vi "Crossover Frame.vi"(8 "error in (no error)":errorcluster, 10 "OSSP_Problem In":refnum<class "OSSP_Problem.lvclass">, 11 "GA in":refnum<class "GA.lvclass">) -> (0 "error out":errorcluster, 2 "OSSP_Problem Out":refnum<class "OSSP_Problem.lvclass">, 3 "GA out":refnum<class "GA.lvclass">)   [LabVIEW 2013, in "GA.lvclass"]
uses:
  GA.lvclass
  OSSP_Problem.lvclass
  GA.lvclass/GA.ctl
  OSSP_Problem.lvclass/OSSP_Problem.ctl
  Controls/MPOX1 Operation Selection Rule.ctl
  Controls/MPOX2 Operation Selection Rule.ctl
  Find Elements not On Other Child.vi
  GA/SubVIS/Remove Duplicates In Array.vi
  GA/SubVIS/OX Crossover Template.vi
  LOX Crossover Template.vi
  Scheduler_Class/Schedule To Operations on Machines.vi
  OSSP_Problem_Class/Getters/Read Processing Times.vi
  Calculate Job and Machine Orders.vi
  Getters/Read Scheduler.vi
  Getters/Read Objective .vi
  MOPX1 Engine.vi
  Scheduler_Class/NonDelay Scheduler/Non Delay Scheduler Engine.vi
  Scheduler_Class/Giffler Thompson Active Schedule Engine.vi
  Scheduler_Class/MyFIFOScheduler.vi
  Scheduler_Class/Job Completion Times.vi
  Scheduler_Class/Prins FIFO Scheduler Methods and Controls/Prins FIFO Scheduler.vi
  Scheduler_Class/Prins FIFO Scheduler Methods and Controls/Methods/Calculate Final Completion Times of Jobs.vi
  OSSP_Problem_Class/Getters/Read Due Dates.vi
  MOPX2 Engine.vi
  Scheduler_Class/Operation to Machine Job Tuple.vi
  Scheduler_Class/Check Other Machines for Schedule Time.vi
  Scheduler_Class/Schedule Job.vi
  Scheduler_Class/Find Gaps on Particular Machine.vi
  Scheduler_Class/Increment Number of Jobs on Machine.vi
  Scheduler_Class/Find Job On Other Machines.vi
  Scheduler_Class/Prins FIFO Scheduler Methods and Controls/Methods/UpdateMachineGaps.vi
  Scheduler_Class/Prins FIFO Scheduler Methods and Controls/Methods/UpdateJobGaps.vi
  Scheduler_Class/Prins FIFO Scheduler Methods and Controls/Methods/Find Intersecting Gaps.vi
  Scheduler_Class/GT Algorithm Find M_ok and J_ok.vi
  Scheduler_Class/Prins FIFO Scheduler Methods and Controls/Methods/Transform to Plain Job and Machine Gaps Array.vi
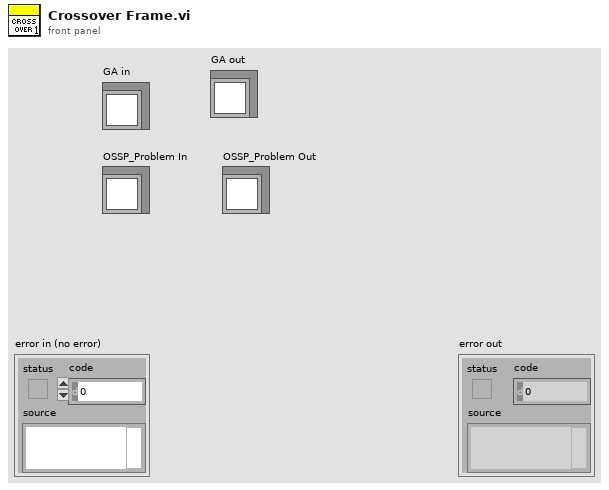
[diagram p1: front panel]
types:
  T1 = typedef "GA.lvclass/MPOX1 Operation Selection Rule.ctl" = enum16{"Min Lateness Job", "Random Job"}
  T2 = typedef "GA.lvclass/MPOX2 Operation Selection Rule.ctl" = enum16{"First Operation of All Jobs", "Random"}
  T3 = typedef "Solution_GA.ctl" = cluster{"Schedule":u16[], "Fitness":u16, "Fitness Valid?":bool}
  T4 = typedef "GA.lvclass/Crossover Type.ctl" = enum16{"One Point Cx", "Two Point Cx", "Ordered Cx (OX)", "Linear Order Cx (LOX)", "PMX", "Uniform PMX", "Cycle Cx", "Specialized Cx", "JO4M Cx", "MPOX1", "MPOX1 Random", "MPOX2", "MPOX2 Random", "SXX"}
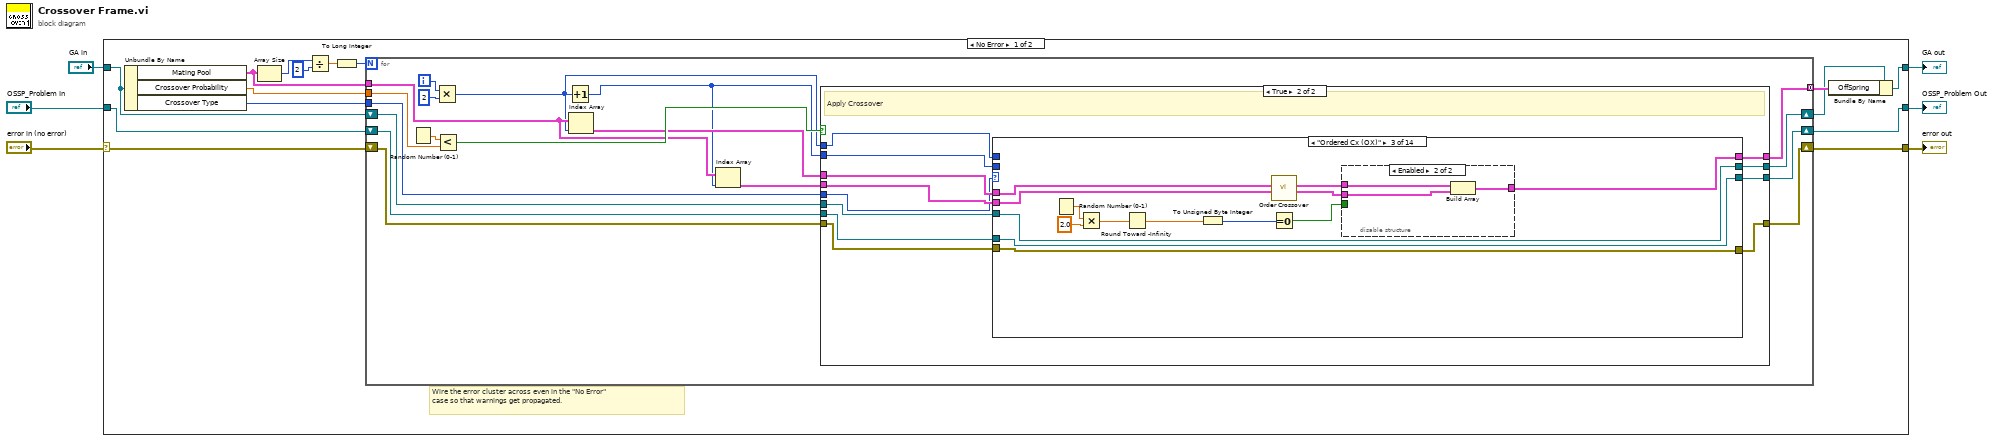
[diagram p0: block diagram]
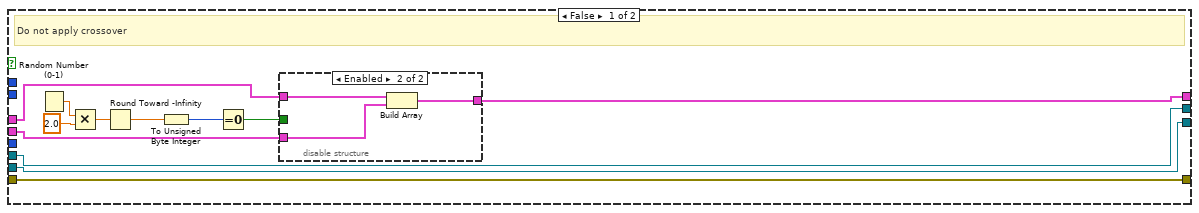
[diagram p2: hidden frame]
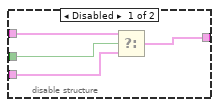
[diagram p3: hidden frame]
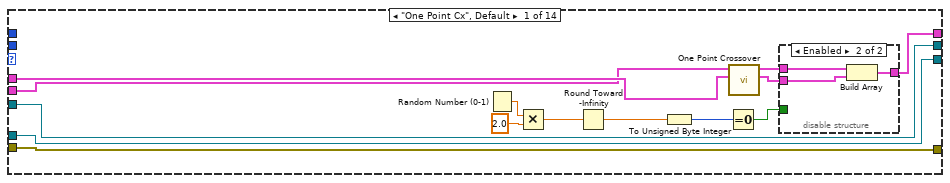
[diagram p4: hidden frame]
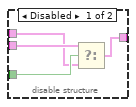
[diagram p5: hidden frame]
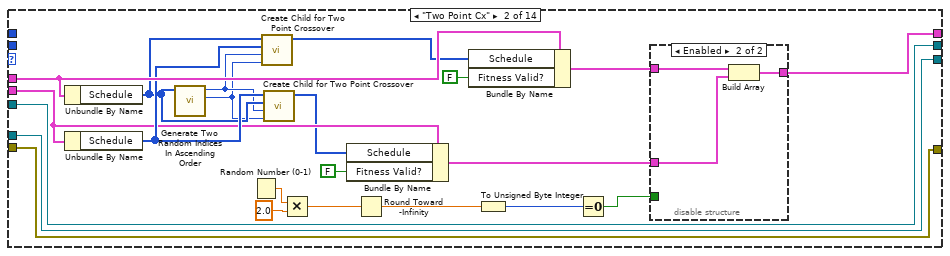
[diagram p6: hidden frame]
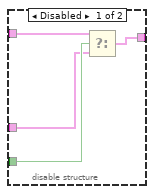
[diagram p7: hidden frame]
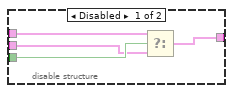
[diagram p8: hidden frame]
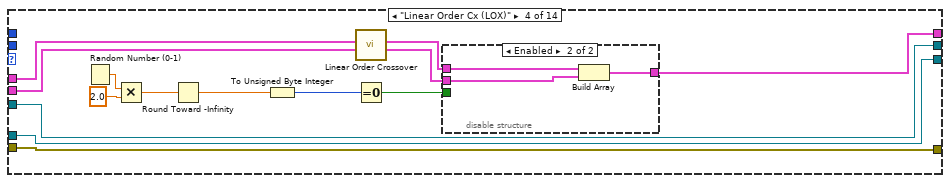
[diagram p9: hidden frame]
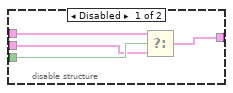
[diagram p10: hidden frame]
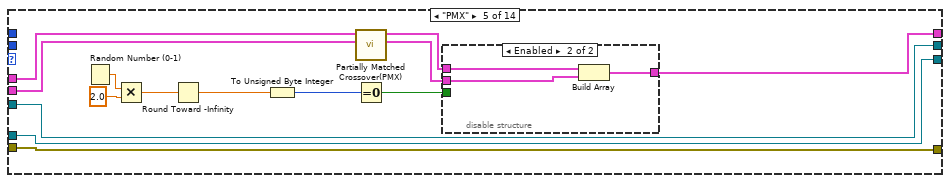
[diagram p11: hidden frame]
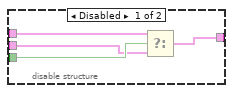
[diagram p12: hidden frame]
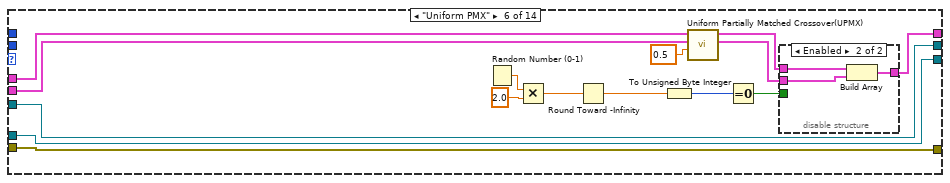
[diagram p13: hidden frame]
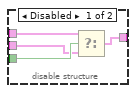
[diagram p14: hidden frame]
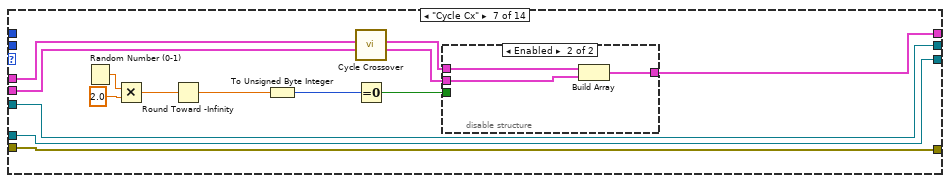
[diagram p15: hidden frame]
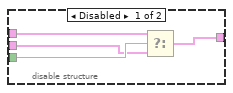
[diagram p16: hidden frame]
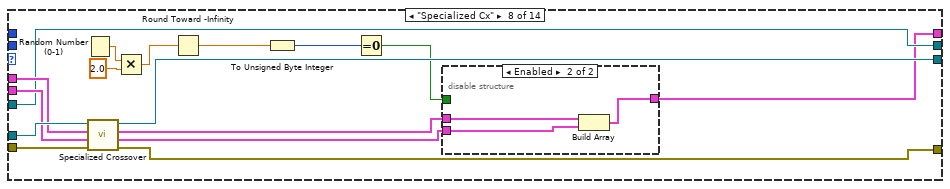
[diagram p17: hidden frame]
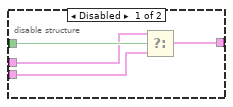
[diagram p18: hidden frame]
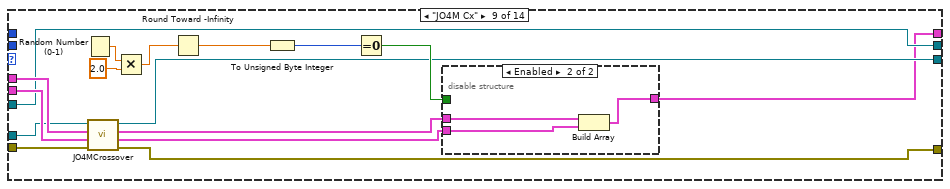
[diagram p19: hidden frame]
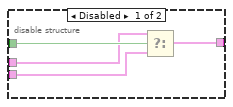
[diagram p20: hidden frame]
diagram:
  n1 = case shown="No Error" "error in (no error)" {
    selector: "error in (no error)" -> [w15 w410]
    tunnel: [w14 w410] -> w5
    tunnel: [w19 w409] -> w3
    tunnel: "GA in" -> [w8 w409]
    tunnel: "OSSP_Problem In" -> [w17 w408]
    tunnel: [w16 w408] -> w1
    frame No Error {
      # "Wire the error cluster across even in the \"No Error\"\ncase so that warnings get propagated."
      n2 = Unbundle By Name(w8) -> ("Mating Pool"=w21:T3[], "Crossover Probability"=w20:dbl, "Crossover Type"=w18:T4)
      n3 = Array Size(array=w21) -> (size(s)=w13:i32)
      n4 = Divide(x=w13, y=2) -> (x/y=w9:dbl)
      n5 = To Long Integer(number=w9) -> (32bit integer=w12:i32)
      n6 = for {
        N: w12 -> [_]
        tunnel: w20 -> [w37]
        tunnel: w18 -> [w30]
        shift-right: [w29] -> w16
        shift-left: w17 -> [w28]
        shift-right: [w26] -> w14
        shift-left: w15 -> [w27]
        tunnel: w21 -> [w33]
        tunnel: [w24] -> w11 mode=concatenating
        shift-right: [w22] -> w7
        shift-left: w8 -> [w23]
        i -> [w39]
        n7 = Random Number (0-1)() -> (number: 0 to 1=w38:dbl)
        n8 = Multiply(x=w39, y=2) -> (x*y=w32:i32)
        n9 = Less?(x=w38, y=w37) -> (x < y?=w36:bool)
        n10 = Increment(x=w32) -> (x+1=w31:i32)
        n11 = Index Array(array=w33, index=w32) -> (element=w35:T3)
        n12 = Index Array(array=w33, index=w31) -> (element=w34:T3)
        n13 = case shown="True" w36 {
          tunnel: w35 -> [w43 w68]
          tunnel: w34 -> [w42 w67]
          tunnel: w32 -> [_ w70]
          tunnel: w31 -> [_ w69]
          tunnel: w30 -> [_ w66]
          tunnel: w28 -> [w51 w65]
          tunnel: [w51 w64] -> w29
          tunnel: w27 -> [w50 w63]
          tunnel: [w50 w62] -> w26
          tunnel: [w40 w61] -> w24
          tunnel: w23 -> [w41 w60]
          tunnel: [w41 w59] -> w22
          frame False {
            # "Do not apply crossover"
            n14 = Random Number (0-1)() -> (number: 0 to 1=w49:dbl)
            n15 = Multiply(x=w49, y=2.0) -> (x*y=w47:dbl)
            n16 = Round Toward -Infinity(1:w47) -> (0:w46:dbl)
            n17 = To Unsigned Byte Integer(number=w46) -> (unsigned 8bit integer=w45:u8)
            n18 = Equal To 0?(x=w45) -> (x = 0?=w44:bool)
            n19 = disable-structure shown="Enabled" {
              disable-tunnel: w44 -> [w55 _]
              disable-tunnel: w43 -> [w54 w58]
              disable-tunnel: w42 -> [w53 w57]
              disable-tunnel: [w52 w56] -> w40
              frame Disabled {
                n20 = Select(t=w54, s=w55, f=w53) -> (s? t:f=w52:T3)
              }
              frame Enabled {
                n21 = Build Array(w58, w57) -> (w56:T3[])
              }
            }
          }
          frame True {
            # "Apply Crossover"
            n22 = case shown="\"Ordered Cx (OX)\"" w66 {
              tunnel: w70 -> [_ _ _ _ _ _ _ _ _ _ _ _ _ _]
              tunnel: w69 -> [_ _ _ _ _ _ _ _ _ _ _ _ _ _]
              tunnel: w68 -> [w84 w111 w132 w153 w173 w194 w217 w237 w259 w289 w316 w344 w370 w400]
              tunnel: w67 -> [w83 w104 w131 w152 w172 w193 w216 w238 w258 w288 w315 w343 w369 w399]
              tunnel: w65 -> [w82 w113 w133 w154 w176 w198 w219 w242 w257 w285 w312 w333 w359 w383]
              tunnel: [w82 w113 w133 w154 w176 w198 w219 w241 w254 w284 w311 w330 w356 w382] -> w64
              tunnel: w63 -> [w81 w112 w134 w155 w175 w197 w218 w240 w256 w292 w319 w345 w371 w386]
              tunnel: [w81 w112 w134 w155 w175 w197 w218 w239 w255 w283 w310 w341 w367 w385] -> w62
              tunnel: [w71 w92 w121 w142 w163 w184 w206 w227 w250 w273 w300 w327 w353 w379] -> w61
              tunnel: w60 -> [w72 w93 w122 w143 w174 w196 w207 w228 w251 w291 w318 w334 w360 w391]
              tunnel: [w72 w93 w122 w143 w174 w196 w207 w228 w251 w290 w317 w334 w360 w391] -> w59
              frame "One Point Cx", Default {
                n23 = Random Number (0-1)() -> (number: 0 to 1=w80:dbl)
                n24 = Multiply(x=w80, y=2.0) -> (x*y=w78:dbl)
                n25 = Round Toward -Infinity(1:w78) -> (0:w77:dbl)
                n26 = To Unsigned Byte Integer(number=w77) -> (unsigned 8bit integer=w76:u8)
                n27 = Equal To 0?(x=w76) -> (x = 0?=w75:bool)
                n28 = call "One Point Crossover.vi"("Parent 1 in"=w84, "Parent 2 in"=w83) -> ("Child 1 out"=w74:T3, "Child 2 Out"=w73:T3)  [unwired: 8 in]
                n29 = disable-structure shown="Enabled" {
                  disable-tunnel: w75 -> [w88 _]
                  disable-tunnel: w74 -> [w87 w89]
                  disable-tunnel: w73 -> [w86 w91]
                  disable-tunnel: [w85 w90] -> w71
                  frame Disabled {
                    n30 = Select(t=w87, s=w88, f=w86) -> (s? t:f=w85:T3)
                  }
                  frame Enabled {
                    n31 = Build Array(w91, w89) -> (w90:T3[])
                  }
                }
              }
              frame "Two Point Cx" {
                n32 = Unbundle By Name(w111) -> ("Schedule"=w107:u16[])
                n33 = Unbundle By Name(w104) -> ("Schedule"=w108:u16[])
                n34 = call "Generate Two Random Indices In Ascending Order.vi"("Schedule"=w107) -> ("Index 2"=w105:i32, "Index 1"=w106:i32)  [unwired: 9 in]
                n35 = Random Number (0-1)() -> (number: 0 to 1=w101:dbl)
                n36 = call "Create Child for Two Point Crossover.vi"("Cut Point Index 2"=w105, "Cut Point Index 1"=w106, "SCH 2"=w108, "SCH 1"=w107) -> ("Child Out"=w110:u16[])  [unwired: 7 in]
                n37 = call "Create Child for Two Point Crossover.vi"("Cut Point Index 2"=w105, "Cut Point Index 1"=w106, "SCH 2"=w107, "SCH 1"=w108) -> ("Child Out"=w103:u16[])  [unwired: 7 in]
                n38 = Multiply(x=w101, y=2.0) -> (x*y=w99:dbl)
                n39 = Bundle By Name(cluster=w104, "Schedule"=w103, "Fitness Valid?"=FALSE) -> (w94:T3)
                n40 = Round Toward -Infinity(1:w99) -> (0:w98:dbl)
                n41 = Bundle By Name(cluster=w111, "Schedule"=w110, "Fitness Valid?"=FALSE) -> (w95:T3)
                n42 = To Unsigned Byte Integer(number=w98) -> (unsigned 8bit integer=w97:u8)
                n43 = Equal To 0?(x=w97) -> (x = 0?=w96:bool)
                n44 = disable-structure shown="Enabled" {
                  disable-tunnel: w96 -> [w117 _]
                  disable-tunnel: w95 -> [w116 w120]
                  disable-tunnel: w94 -> [w115 w119]
                  disable-tunnel: [w114 w118] -> w92
                  frame Disabled {
                    n45 = Select(t=w116, s=w117, f=w115) -> (s? t:f=w114:T3)
                  }
                  frame Enabled {
                    n46 = Build Array(w120, w119) -> (w118:T3[])
                  }
                }
              }
              frame "Ordered Cx (OX)" {
                n47 = Random Number (0-1)() -> (number: 0 to 1=w130:dbl)
                n48 = Multiply(x=w130, y=2.0) -> (x*y=w128:dbl)
                n49 = Round Toward -Infinity(1:w128) -> (0:w127:dbl)
                n50 = To Unsigned Byte Integer(number=w127) -> (unsigned 8bit integer=w126:u8)
                n51 = call "Order Crossover.vi"("Parent 2"=w131, "Parent 1"=w132) -> ("Child 2"=w123:T3, "Child 1"=w124:T3)  [unwired: 8 in]
                n52 = Equal To 0?(x=w126) -> (x = 0?=w125:bool)
                n53 = disable-structure shown="Enabled" {
                  disable-tunnel: w125 -> [w138 _]
                  disable-tunnel: w124 -> [w137 w141]
                  disable-tunnel: w123 -> [w136 w140]
                  disable-tunnel: [w135 w139] -> w121
                  frame Disabled {
                    n54 = Select(t=w137, s=w138, f=w136) -> (s? t:f=w135:T3)
                  }
                  frame Enabled {
                    n55 = Build Array(w141, w140) -> (w139:T3[])
                  }
                }
              }
              frame "Linear Order Cx (LOX)" {
                n56 = Random Number (0-1)() -> (number: 0 to 1=w151:dbl)
                n57 = Multiply(x=w151, y=2.0) -> (x*y=w149:dbl)
                n58 = Round Toward -Infinity(1:w149) -> (0:w148:dbl)
                n59 = To Unsigned Byte Integer(number=w148) -> (unsigned 8bit integer=w147:u8)
                n60 = call "Linear Order Crossover.vi"("Parent 2"=w152, "Parent 1"=w153) -> ("Child 2"=w144:T3, "Child 1"=w145:T3)  [unwired: 8 in]
                n61 = Equal To 0?(x=w147) -> (x = 0?=w146:bool)
                n62 = disable-structure shown="Enabled" {
                  disable-tunnel: w146 -> [w159 _]
                  disable-tunnel: w145 -> [w158 w162]
                  disable-tunnel: w144 -> [w157 w161]
                  disable-tunnel: [w156 w160] -> w142
                  frame Disabled {
                    n63 = Select(t=w158, s=w159, f=w157) -> (s? t:f=w156:T3)
                  }
                  frame Enabled {
                    n64 = Build Array(w162, w161) -> (w160:T3[])
                  }
                }
              }
              frame "PMX" {
                n65 = Random Number (0-1)() -> (number: 0 to 1=w171:dbl)
                n66 = Multiply(x=w171, y=2.0) -> (x*y=w169:dbl)
                n67 = Round Toward -Infinity(1:w169) -> (0:w168:dbl)
                n68 = To Unsigned Byte Integer(number=w168) -> (unsigned 8bit integer=w167:u8)
                n69 = call "Partially Matched Crossover(PMX).vi"("Ind 2"=w172, "Ind 1"=w173) -> ("Child 2"=w164:T3, "Child 1"=w165:T3)  [unwired: 8 in]
                n70 = Equal To 0?(x=w167) -> (x = 0?=w166:bool)
                n71 = disable-structure shown="Enabled" {
                  disable-tunnel: w166 -> [w180 _]
                  disable-tunnel: w165 -> [w179 w183]
                  disable-tunnel: w164 -> [w178 w182]
                  disable-tunnel: [w177 w181] -> w163
                  frame Disabled {
                    n72 = Select(t=w179, s=w180, f=w178) -> (s? t:f=w177:T3)
                  }
                  frame Enabled {
                    n73 = Build Array(w183, w182) -> (w181:T3[])
                  }
                }
              }
              frame "Uniform PMX" {
                n74 = Random Number (0-1)() -> (number: 0 to 1=w192:dbl)
                n75 = Multiply(x=w192, y=2.0) -> (x*y=w190:dbl)
                n76 = Round Toward -Infinity(1:w190) -> (0:w189:dbl)
                n77 = To Unsigned Byte Integer(number=w189) -> (unsigned 8bit integer=w188:u8)
                n78 = call "Uniform Partially Matched Crossover(UPMX).vi"("indpb"=0.5, "Ind 2"=w193, "Ind 1"=w194) -> ("Child 2"=w185:T3, "Child 1"=w186:T3)  [unwired: 7 in]
                n79 = Equal To 0?(x=w188) -> (x = 0?=w187:bool)
                n80 = disable-structure shown="Enabled" {
                  disable-tunnel: w187 -> [w202 _]
                  disable-tunnel: w186 -> [w201 w205]
                  disable-tunnel: w185 -> [w200 w204]
                  disable-tunnel: [w199 w203] -> w184
                  frame Disabled {
                    n81 = Select(t=w201, s=w202, f=w200) -> (s? t:f=w199:T3)
                  }
                  frame Enabled {
                    n82 = Build Array(w205, w204) -> (w203:T3[])
                  }
                }
              }
              frame "Cycle Cx" {
                n83 = Random Number (0-1)() -> (number: 0 to 1=w215:dbl)
                n84 = Multiply(x=w215, y=2.0) -> (x*y=w213:dbl)
                n85 = Round Toward -Infinity(1:w213) -> (0:w212:dbl)
                n86 = To Unsigned Byte Integer(number=w212) -> (unsigned 8bit integer=w211:u8)
                n87 = call "Cycle Crossover.vi"("Parent 2"=w216, "Parent 1"=w217) -> ("Child 2"=w208:T3, "Child 1"=w209:T3)  [unwired: 8 in]
                n88 = Equal To 0?(x=w211) -> (x = 0?=w210:bool)
                n89 = disable-structure shown="Enabled" {
                  disable-tunnel: w210 -> [w223 _]
                  disable-tunnel: w209 -> [w222 w226]
                  disable-tunnel: w208 -> [w221 w225]
                  disable-tunnel: [w220 w224] -> w206
                  frame Disabled {
                    n90 = Select(t=w222, s=w223, f=w221) -> (s? t:f=w220:T3)
                  }
                  frame Enabled {
                    n91 = Build Array(w226, w225) -> (w224:T3[])
                  }
                }
              }
              frame "Specialized Cx" {
                n92 = Random Number (0-1)() -> (number: 0 to 1=w236:dbl)
                n93 = call "Specialized Crossover.vi"("error in (no error)"=w240, "Parent 2"=w238, "Parent 1"=w237, "OSSP_Problem in"=w242) -> ("error out"=w239:errorcluster, "Child 2"=w229:T3, "Child 1"=w230:T3, "OSSP_Problem out"=w241:refnum<class "OSSP_Problem.lvclass">)  [unwired: 4 in]
                n94 = Multiply(x=w236, y=2.0) -> (x*y=w234:dbl)
                n95 = Round Toward -Infinity(1:w234) -> (0:w233:dbl)
                n96 = To Unsigned Byte Integer(number=w233) -> (unsigned 8bit integer=w232:u8)
                n97 = Equal To 0?(x=w232) -> (x = 0?=w231:bool)
                n98 = disable-structure shown="Enabled" {
                  disable-tunnel: w231 -> [w246 _]
                  disable-tunnel: w230 -> [w245 w249]
                  disable-tunnel: w229 -> [w244 w248]
                  disable-tunnel: [w243 w247] -> w227
                  frame Disabled {
                    n99 = Select(t=w245, s=w246, f=w244) -> (s? t:f=w243:T3)
                  }
                  frame Enabled {
                    n100 = Build Array(w249, w248) -> (w247:T3[])
                  }
                }
              }
              frame "JO4M Cx" {
                n101 = Random Number (0-1)() -> (number: 0 to 1=w265:dbl)
                n102 = call "JO4MCrossover.vi"("error in (no error)"=w256, "Parent 2"=w258, "Parent 1"=w259, "OSSP_Problem in"=w257) -> ("error out"=w255:errorcluster, "Child 2"=w252:T3, "Child 1"=w253:T3, "OSSP_Problem out"=w254:refnum<class "OSSP_Problem.lvclass">)  [unwired: 4 in]
                n103 = Multiply(x=w265, y=2.0) -> (x*y=w263:dbl)
                n104 = Round Toward -Infinity(1:w263) -> (0:w262:dbl)
                n105 = To Unsigned Byte Integer(number=w262) -> (unsigned 8bit integer=w261:u8)
                n106 = Equal To 0?(x=w261) -> (x = 0?=w260:bool)
                n107 = disable-structure shown="Enabled" {
                  disable-tunnel: w260 -> [w269 _]
                  disable-tunnel: w253 -> [w268 w272]
                  disable-tunnel: w252 -> [w267 w271]
                  disable-tunnel: [w266 w270] -> w250
                  frame Disabled {
                    n108 = Select(t=w268, s=w269, f=w267) -> (s? t:f=w266:T3)
                  }
                  frame Enabled {
                    n109 = Build Array(w272, w271) -> (w270:T3[])
                  }
                }
              }
              frame "MPOX1" {
                n110 = Unbundle By Name(w289) -> ("Schedule"=w287:u16[])
                n111 = Unbundle By Name(w288) -> ("Schedule"=w286:u16[])
                n112 = Random Number (0-1)() -> (number: 0 to 1=w282:dbl)
                n113 = Multiply(x=w282, y=2.0) -> (x*y=w280:dbl)
                n114 = Round Toward -Infinity(1:w280) -> (0:w279:dbl)
                n115 = To Unsigned Byte Integer(number=w279) -> (unsigned 8bit integer=w278:u8)
                n116 = call "MOPX1 Crossover.vi"("Job Selection Rule"=MPOX1_Operation_Selection_Rule."Min Lateness Job", "Parent 1 Schedule"=w287, "error in (no error)"=w292, "Parent 2 Schedule"=w286, "OSSP_Problem In"=w285, "GA in"=w291) -> ("error out"=w283:errorcluster, "Child 1"=w276:T3, "OSSP_Problem out"=w284:refnum<class "OSSP_Problem.lvclass">, "GA out"=w290:refnum<class "GA.lvclass">, "Child 2"=w275:T3)  [unwired: 1 in]
                n117 = Equal To 0?(x=w278) -> (x = 0?=w277:bool)
                n118 = disable-structure shown="Enabled" {
                  disable-tunnel: w277 -> [w296 _]
                  disable-tunnel: w276 -> [w295 w299]
                  disable-tunnel: w275 -> [w294 w298]
                  disable-tunnel: [w293 w297] -> w273
                  frame Disabled {
                    n119 = Select(t=w295, s=w296, f=w294) -> (s? t:f=w293:T3)
                  }
                  frame Enabled {
                    n120 = Build Array(w299, w298) -> (w297:T3[])
                  }
                }
              }
              frame "MPOX1 Random" {
                n121 = Unbundle By Name(w316) -> ("Schedule"=w314:u16[])
                n122 = Unbundle By Name(w315) -> ("Schedule"=w313:u16[])
                n123 = Random Number (0-1)() -> (number: 0 to 1=w309:dbl)
                n124 = Multiply(x=w309, y=2.0) -> (x*y=w307:dbl)
                n125 = Round Toward -Infinity(1:w307) -> (0:w306:dbl)
                n126 = To Unsigned Byte Integer(number=w306) -> (unsigned 8bit integer=w305:u8)
                n127 = call "MOPX1 Crossover.vi"("Job Selection Rule"=MPOX1_Operation_Selection_Rule."Random Job", "Parent 1 Schedule"=w314, "error in (no error)"=w319, "Parent 2 Schedule"=w313, "OSSP_Problem In"=w312, "GA in"=w318) -> ("error out"=w310:errorcluster, "Child 1"=w303:T3, "OSSP_Problem out"=w311:refnum<class "OSSP_Problem.lvclass">, "GA out"=w317:refnum<class "GA.lvclass">, "Child 2"=w302:T3)  [unwired: 1 in]
                n128 = Equal To 0?(x=w305) -> (x = 0?=w304:bool)
                n129 = disable-structure shown="Enabled" {
                  disable-tunnel: w304 -> [w323 _]
                  disable-tunnel: w303 -> [w322 w326]
                  disable-tunnel: w302 -> [w321 w325]
                  disable-tunnel: [w320 w324] -> w300
                  frame Disabled {
                    n130 = Select(t=w322, s=w323, f=w321) -> (s? t:f=w320:T3)
                  }
                  frame Enabled {
                    n131 = Build Array(w326, w325) -> (w324:T3[])
                  }
                }
              }
              frame "MPOX2" {
                n132 = Unbundle By Name(w344) -> ("Schedule"=w332:u16[])
                n133 = Unbundle By Name(w343) -> ("Schedule"=w342:u16[])
                n134 = Random Number (0-1)() -> (number: 0 to 1=w340:dbl)
                n135 = Multiply(x=w340, y=2.0) -> (x*y=w338:dbl)
                n136 = Round Toward -Infinity(1:w338) -> (0:w337:dbl)
                n137 = To Unsigned Byte Integer(number=w337) -> (unsigned 8bit integer=w336:u8)
                n138 = call "MOPX2 Crossover.vi"("Operation Selection"=MPOX2_Operation_Selection_Rule."First Operation of All Jobs", "error in (no error)"=w345, "Parent 2 Schedule"=w342, "Parent 1 Schedule"=w332, "OSSP_Problem In"=w333) -> ("error out"=w341:errorcluster, "Child 2"=w328:T3, "Child 1"=w329:T3, "OSSP_Problem out"=w330:refnum<class "OSSP_Problem.lvclass">)  [unwired: 3 in]
                n139 = Equal To 0?(x=w336) -> (x = 0?=w335:bool)
                n140 = disable-structure shown="Enabled" {
                  disable-tunnel: w335 -> [w349 _]
                  disable-tunnel: w329 -> [w348 w352]
                  disable-tunnel: w328 -> [w347 w351]
                  disable-tunnel: [w346 w350] -> w327
                  frame Disabled {
                    n141 = Select(t=w348, s=w349, f=w347) -> (s? t:f=w346:T3)
                  }
                  frame Enabled {
                    n142 = Build Array(w352, w351) -> (w350:T3[])
                  }
                }
              }
              frame "MPOX2 Random" {
                n143 = Unbundle By Name(w370) -> ("Schedule"=w358:u16[])
                n144 = Unbundle By Name(w369) -> ("Schedule"=w368:u16[])
                n145 = Random Number (0-1)() -> (number: 0 to 1=w366:dbl)
                n146 = Multiply(x=w366, y=2.0) -> (x*y=w364:dbl)
                n147 = Round Toward -Infinity(1:w364) -> (0:w363:dbl)
                n148 = To Unsigned Byte Integer(number=w363) -> (unsigned 8bit integer=w362:u8)
                n149 = call "MOPX2 Crossover.vi"("Operation Selection"=MPOX2_Operation_Selection_Rule."Random", "error in (no error)"=w371, "Parent 2 Schedule"=w368, "Parent 1 Schedule"=w358, "OSSP_Problem In"=w359) -> ("error out"=w367:errorcluster, "Child 2"=w354:T3, "Child 1"=w355:T3, "OSSP_Problem out"=w356:refnum<class "OSSP_Problem.lvclass">)  [unwired: 3 in]
                n150 = Equal To 0?(x=w362) -> (x = 0?=w361:bool)
                n151 = disable-structure shown="Enabled" {
                  disable-tunnel: w361 -> [w375 _]
                  disable-tunnel: w355 -> [w374 w378]
                  disable-tunnel: w354 -> [w373 w377]
                  disable-tunnel: [w372 w376] -> w353
                  frame Disabled {
                    n152 = Select(t=w374, s=w375, f=w373) -> (s? t:f=w372:T3)
                  }
                  frame Enabled {
                    n153 = Build Array(w378, w377) -> (w376:T3[])
                  }
                }
              }
              frame "SXX" {
                n154 = Unbundle By Name(w400) -> ("Schedule"=w390:u16[])
                n155 = Unbundle By Name(w399) -> ("Schedule"=w398:u16[])
                n156 = call "Read Number of Machines.vi"("error in (no error)"=w386, "OSSP_Problem in"=w383) -> ("error out"=w387:errorcluster, "Number of Machines"=w381:i32, "OSSP_Problem out"=w384:refnum<class "OSSP_Problem.lvclass">)  [unwired: 7 in]
                n157 = call "Read Number of Jobs.vi"("error in (no error)"=w387, "OSSP_Problem in"=w384) -> ("error out"=w385:errorcluster, "Number of Jobs"=w380:i32, "OSSP_Problem out"=w382:refnum<class "OSSP_Problem.lvclass">)  [unwired: 7 in]
                n158 = Random Number (0-1)() -> (number: 0 to 1=w397:dbl)
                n159 = Multiply(x=w397, y=2.0) -> (x*y=w395:dbl)
                n160 = call "Subsequence Exchange Crossover(SXX).vi"("Number of Jobs"=w380, "Number of Machines"=w381, "Schedule 2"=w390, "Schedule 1"=w398) -> ("Child 2"=w388:T3, "Child 1"=w389:T3)  [unwired: 6 in]
                n161 = Round Toward -Infinity(1:w395) -> (0:w394:dbl)
                n162 = To Unsigned Byte Integer(number=w394) -> (unsigned 8bit integer=w393:u8)
                n163 = Equal To 0?(x=w393) -> (x = 0?=w392:bool)
                n164 = disable-structure shown="Enabled" {
                  disable-tunnel: w392 -> [w404 _]
                  disable-tunnel: w389 -> [w403 w407]
                  disable-tunnel: w388 -> [w402 w406]
                  disable-tunnel: [w401 w405] -> w379
                  frame Disabled {
                    n165 = Select(t=w403, s=w404, f=w402) -> (s? t:f=w401:T3)
                  }
                  frame Enabled {
                    n166 = Build Array(w407, w406) -> (w405:T3[])
                  }
                }
              }
            }
          }
        }
      }
      n167 = Bundle By Name(cluster=w7, "OffSpring"=w11) -> (w19:refnum<class "GA.lvclass">)
    }
    frame Error {
    }
  }
  "error out" <- w5
  "GA out" <- w3
  "OSSP_Problem Out" <- w1
